vi "resonant image correction.vi"(8 "shift index":i32(slide) scale=0.0..130.0, 10 "pixels per period (2pi, 2 lines)":dbl=1560.0, 11 "x pixels":i32=512) -> (2 "histogram cumsum":dbl[](graph), 3 "histogram pixels to avg":dbl[](graph))   [LabVIEW 2012]
uses:
  <vilib>/Analysis/NI_AALBase.lvlib
panel:
  out "histogram cumsum 2":dbl[](graph)
  out "Histogram: h(x)":i32[](array[numeric])
  out "Array":i32[](array[numeric])
  out "pixels per line":dbl
  out "Histogram Graph":T1(graph)
  out "Waveform Graph":dbl[](graph)
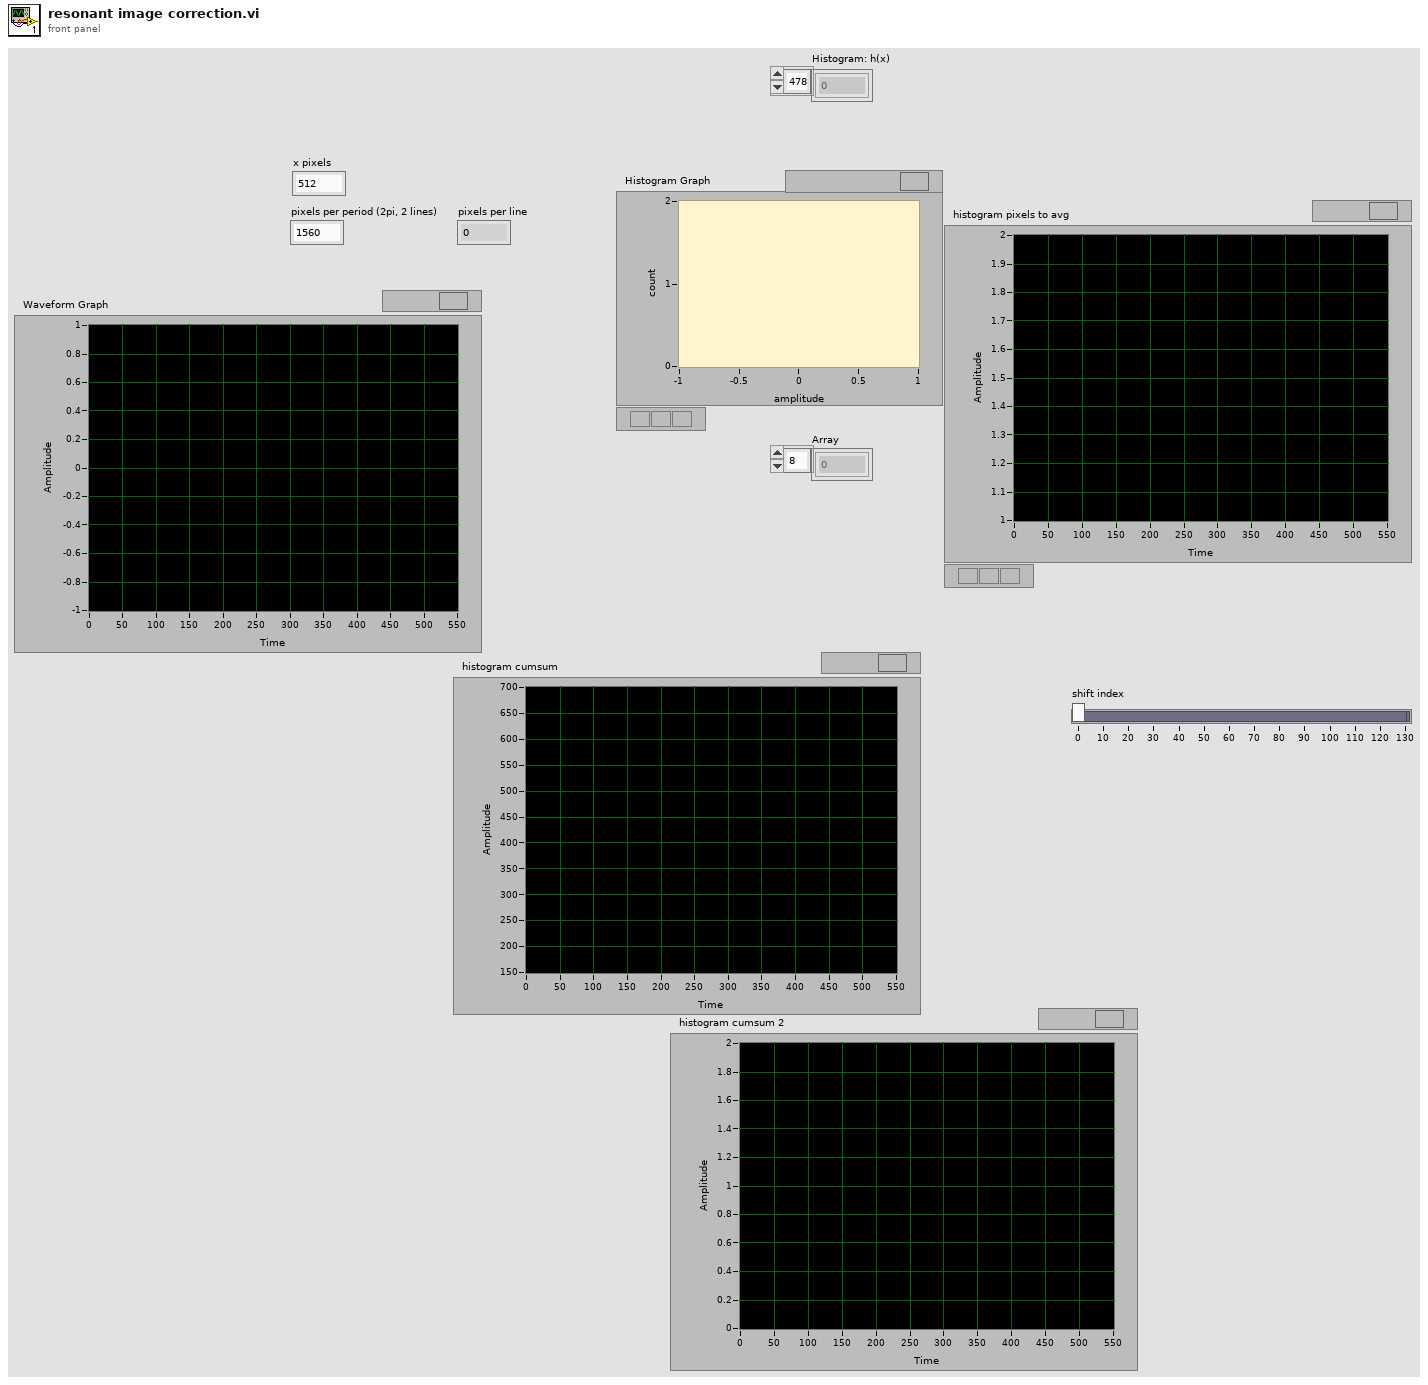
[diagram p1: front panel]
types:
  T1 = cluster{"X Values":dbl[], "Histogram: h(x)":i32[]}
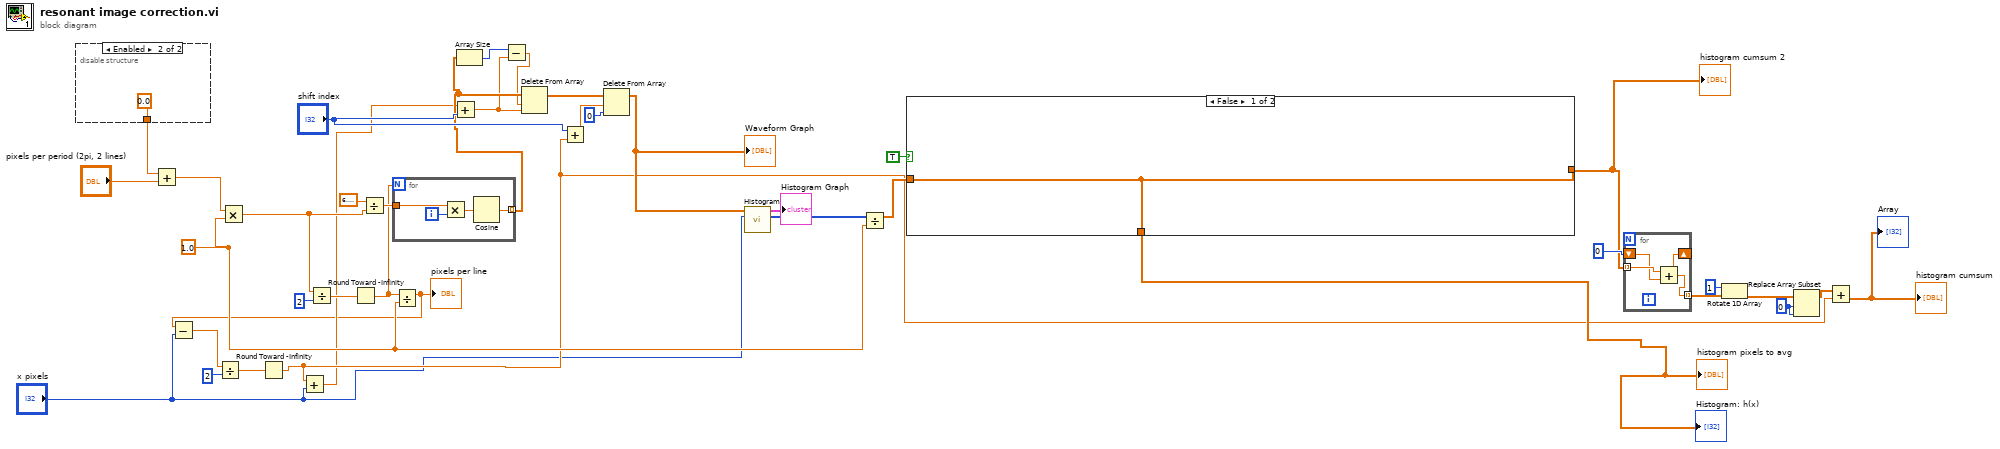
[diagram p0: block diagram]
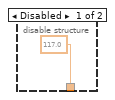
[diagram p2: hidden frame]
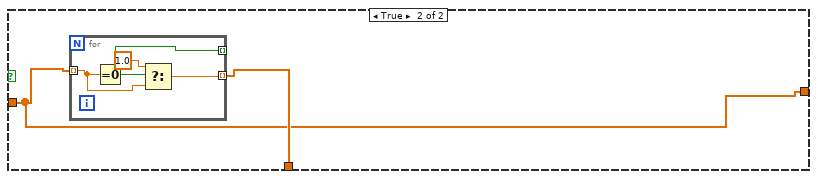
[diagram p3: hidden frame]
diagram:
  w26 = 1.0 ("y")
  w28 = 0 ("index")
  n1 = disable-structure shown="Enabled" {
    disable-tunnel: [117.0 ("x") 0.0 ("x")] -> w9
    frame Disabled {
    }
    frame Enabled {
    }
  }
  n2 = Add(x=w9, y="pixels per period (2pi, 2 lines)") -> (x+y=w8:dbl)
  n3 = Multiply(x=w8, y=w26) -> (x*y=w27:dbl)
  n4 = Divide(x=w27, y=2 ("two lines per cycle")) -> (x/y=w36:dbl)
  n5 = Round Toward -Infinity(1:w36) -> (0:w33:dbl)
  n6 = Divide(x=6.283185307179586, y=w27) -> (x/y=w38:dbl)
  n7 = for {
    N: w33 -> [_]
    tunnel: w38 -> [w44]
    tunnel: [w42] -> w13 mode=indexing
    i -> [w43]
    n8 = Multiply(x=w44, y=w43) -> (x*y=w45:dbl)
    n9 = Cosine(x=w45) -> (cos(x)=w42:dbl)
  }
  n10 = Divide(x=w33, y=w26) -> (x/y=w1:dbl)
  "pixels per line" <- w1
  n11 = Subtract(x=w1, y="x pixels") -> (x-y=w5:dbl)
  n12 = Divide(x=w5, y=2 ("two lines per cycle")) -> (x/y=w6:dbl)
  n13 = Round Toward -Infinity(1:w6) -> (0:w4:dbl)
  n14 = Add(x=w4, y="x pixels") -> (x+y=w2:dbl)
  n15 = Add(x=w2, y="shift index") -> (x+y=w11:dbl)
  n16 = Array Size(array=w13) -> (size(s)=w12:i32)
  n17 = Subtract(x=w12, y=w11) -> (x-y=w10:dbl)
  n18 = Delete From Array(array=w13, length=w10, index=w11) -> (array with subset deleted=w18:dbl[])  [unwired: 1 out]
  n19 = Add(x="shift index", y=w4) -> (x+y=w22:dbl)
  n20 = Delete From Array(array=w18, length=w22, index=0 ("disabled index (col)")) -> (array with subset deleted=w17:dbl[])  [unwired: 1 out]
  "Waveform Graph" <- w17
  n21 = call <vilib>:"Histogram.vi"("intervals"="x pixels", "X"=w17) -> ("Histogram: h(x)"=w31:i32[], "Histogram Graph"=→"Histogram Graph":T1)  [unwired: 6 in, 2 out]
  n22 = Divide(x=w31, y=w26) -> (x/y=w24:dbl[])
  n23 = case shown="False" TRUE {
    tunnel: w24 -> [w46 w47]
    tunnel: [w46 w47] -> w14
    tunnel: [w46 w48] -> w16
    frame False {
    }
    frame True {
      n24 = for {
        tunnel: w47 -> [w51] mode=indexing
        tunnel: [w50] -> w48 mode=indexing
        tunnel: [w49] -> _ mode=indexing
        n25 = Equal To 0?(x=w51) -> (x = 0?=w49:bool)
        n26 = Select(t=1.0, s=w49, f=w51) -> (s? t:f=w50:dbl)
      }
    }
  }
  "histogram pixels to avg" <- w16
  "Histogram: h(x)" <- w16
  "histogram cumsum 2" <- w14
  n27 = for {
    tunnel: w14 -> [w55] mode=indexing
    shift-right: [w53] -> _
    shift-left: 0 -> [w54]
    tunnel: [w53] -> w32 mode=indexing
    n28 = Add(x=w55, y=w54) -> (x+y=w53:dbl)
  }
  n29 = Rotate 1D Array(1:w32, 2:1 ("n")) -> (0:w30:dbl[])
  n30 = Replace Array Subset(array=w30, new element=w28, index=w28) -> (w19:dbl[])
  n31 = Add(x=w19, y=w4) -> (x+y=→"histogram cumsum" →"Array":dbl[])
